vi "FGV_Initialization.vi"(8 "error in (no error)":errorcluster) -> (0 "error out":errorcluster)   [LabVIEW 2025]
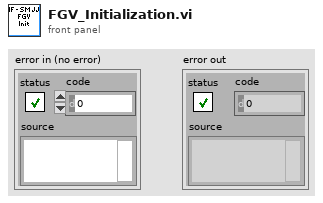
[diagram p1: front panel]
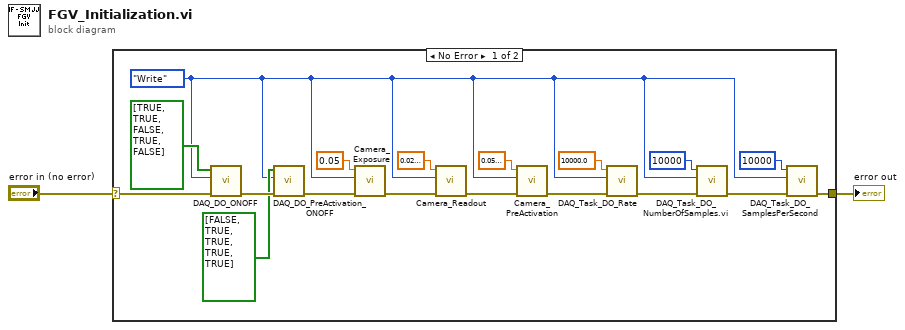
[diagram p0: block diagram]
diagram:
  n1 = case shown="No Error" "error in (no error)" {
    selector: "error in (no error)" -> [w11 w21]
    tunnel: [w4 w21] -> w2
    frame No Error {
      w6 = enum16{"Write", "Read"}."Write" ("Action")
      n2 = call "DAQ_DO_ONOFF.vi"("error in"=w11, "Action"=w6, "DO | ON/OFF"=bool[] [TRUE, TRUE, FALSE, TRUE, FALSE]) -> ("error out"=w19:errorcluster)  [unwired: 7 in, 1 out]
      n3 = call "DAQ_DO_PreActivation_ONOFF.vi"("error in"=w19, "Action"=w6, "DO | PreActivation ON/OFF"=bool[] [FALSE, TRUE, TRUE, TRUE, TRUE] ("DO | PreActivation")) -> ("error out"=w20:errorcluster)  [unwired: 7 in, 1 out]
      n4 = call "Camera_Exposure.vi"("error in"=w20, "Action"=w6, "Exposure (s)"=0.05 ("Exposure time (s)")) -> ("error out"=w15:errorcluster)  [unwired: 7 in, 1 out]
      n5 = call "Camera_Readout.vi"("error in"=w15, "Action"=w6, "Camera_Readout"=0.020000000000000018 ("Readout time (s)")) -> ("error out"=w17:errorcluster)  [unwired: 7 in, 1 out]
      n6 = call "Camera_PreActivation.vi"("error in"=w17, "Action"=w6, "Camera_PreActivation"=0.050000000000000044 ("Pre-activation time (s)")) -> ("error out"=w9:errorcluster)  [unwired: 7 in, 1 out]
      n7 = call "DAQ_Task_DO_Rate.vi"("error in"=w9, "Action"=w6, "DO_Rate"=10000.0) -> ("error out"=w10:errorcluster)  [unwired: 7 in, 1 out]
      n8 = call "DAQ_Task_DO_NumberOfSamples.vi.vi"("error in"=w10, "Action"=w6, "Samples"=10000) -> ("error out"=w5:errorcluster)  [unwired: 7 in, 1 out]
      n9 = call "DAQ_Task_DO_SamplesPerSecond.vi"("error in"=w5, "Action"=w6, "DO_Task_SamplesPerSec"=u32 10000) -> ("error out"=w4:errorcluster)  [unwired: 7 in, 1 out]
    }
    frame Error {
    }
  }
  "error out" <- w2
